vi "Write Motors.vi"(8 "error in (no error)":errorcluster, 10 "Motors":refnum<class "SGDV Motor.lvclass">[](array[class]), 11 "SGDV FPGA Target in":refnum<class "SGDV FPGA Target.lvclass">) -> (0 "error out":errorcluster, 3 "SGDV FPGA Target out":refnum<class "SGDV FPGA Target.lvclass">)   [LabVIEW 2013, in "SGDV_Ctrl_v13_lib.lvlib" / "SGDV FPGA Target.lvclass"]
uses:
  SGDV FPGA Target.lvclass
  SGDV_Ctrl_Class/SGDV Motor.lvclass
  SGDV FPGA Target.lvclass/SGDV FPGA Target.ctl
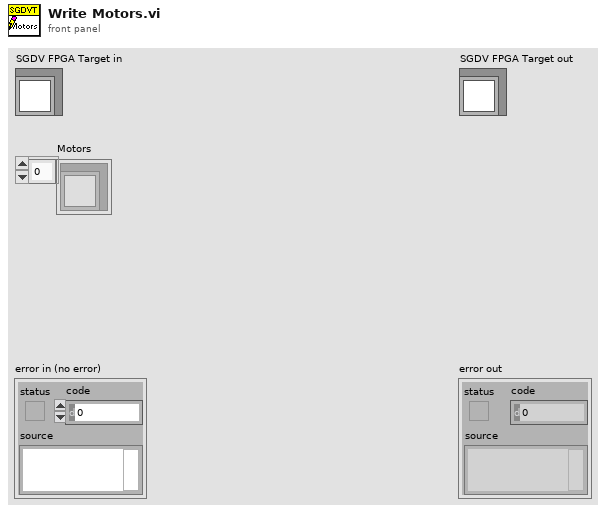
[diagram p1: front panel]
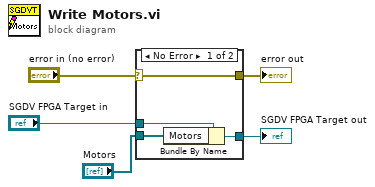
[diagram p0: block diagram]
diagram:
  n1 = case shown="No Error" "error in (no error)" {
    selector: "error in (no error)" -> [w9 w10]
    tunnel: [w9 w10] -> w4
    tunnel: [w7 w11] -> w2
    tunnel: "SGDV FPGA Target in" -> [w8 w11]
    tunnel: "Motors" -> [w6 _]
    frame No Error {
      n2 = Bundle By Name(cluster=w8, "Motors"=w6) -> (w7:refnum<class "SGDV FPGA Target.lvclass">)
    }
    frame Error {
    }
  }
  "error out" <- w4
  "SGDV FPGA Target out" <- w2
